vi "Get Object Pointer.vi"(11 "TreeNodeArray in":refnum<class "TreeNodeArray.lvclass">) -> (1 "Object Pointer":i64, 2 "Assigned object pointer?":bool, 3 "TreeNodeArray out":refnum<class "TreeNodeArray.lvclass">)   [LabVIEW 2012, in "MDSplus.lvlib" / "TreeNodeArray.lvclass"]
uses:
  <vilib>/MDSplus/Classes/TreeNodeArray_Class/TreeNodeArray.lvclass
  <vilib>/MDSplus/Classes/TreeNodeArray_Class/TreeNodeArray.lvclass/TreeNodeArray.ctl
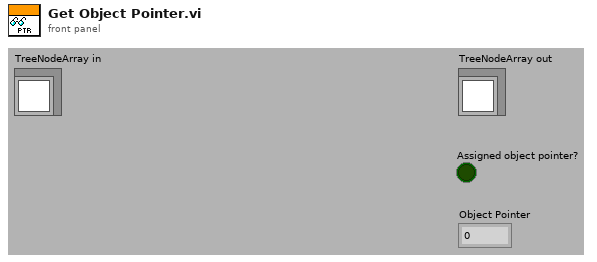
[diagram p1: front panel]
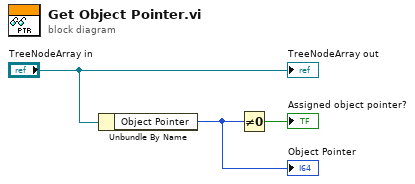
[diagram p0: block diagram]
diagram:
  n1 = Unbundle By Name("TreeNodeArray in") -> ("Object Pointer"=w1:i64)
  "Object Pointer" <- w1
  n2 = Not Equal To 0?(x=w1) -> (x != 0?=→"Assigned object pointer?":bool)
  "TreeNodeArray out" <- "TreeNodeArray in"
